vi "testUManagerReadWriteTXT.vi"() -> ()   [LabVIEW 2021]
panel:
  in  "numImg":dbl
  in  "expTime":dbl
  in  "start":dbl
  in  "file path AcqSettings":path=path "C:/neoDiag/MrAnderson/uManagerBSH/AcqSetings.txt"
  out "error out":errorcluster
  in  "error in":errorcluster
  in  "file path labViewCom":path=path "C:/neoDiag/MrAnderson/uManagerBSH/labViewCom.txt"
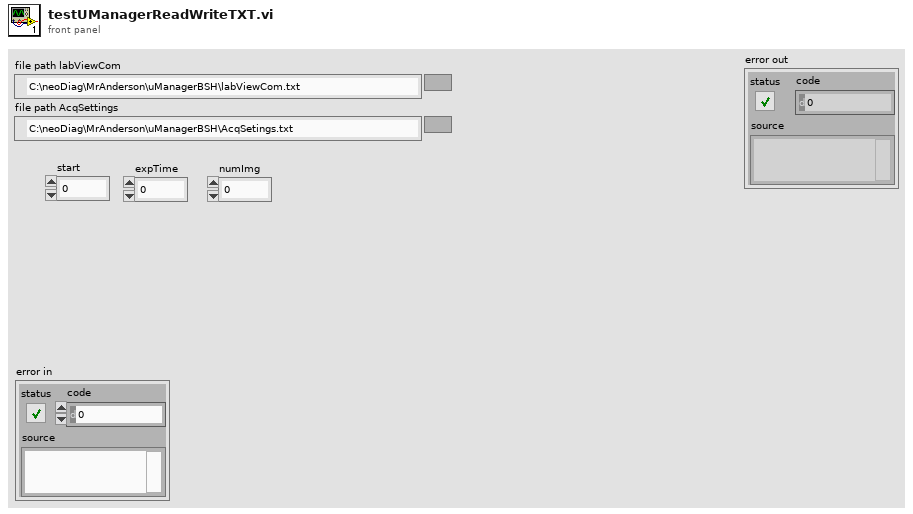
[diagram p1: front panel]
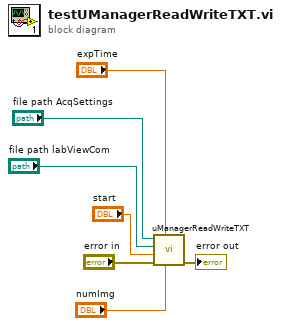
[diagram p0: block diagram]
diagram:
  n1 = call "uManagerReadWriteTXT.vi"("numImg"="numImg", "expTime"="expTime", "error in (no error)"="error in", "start"="start", "file path labViewCom"="file path labViewCom", "file path AcqSettings"="file path AcqSettings") -> ("error out"=→"error out":errorcluster)  [unwired: 3 in]
